vi "Ic_CylindricalLens.vi"(6 "Pixel Pitch 0:20um_or_ 1:12.5um":u8, 7 "Mode Select":enum32{"Row", "Column"}(radio), 8 "error in (no error)":errorcluster, 9 "Wave Length / nm":u32=1064, 10 "Cylindrical Focus / mm":i32=5000, 11 "2D array in (LCOS size buf)":u8[][](array[numeric])) -> (0 "error out":errorcluster, 3 "2D array out":u8[][](array[numeric]))   [LabVIEW 2016]
uses:
  SLM_Control_VI_source/Image_Control.dll
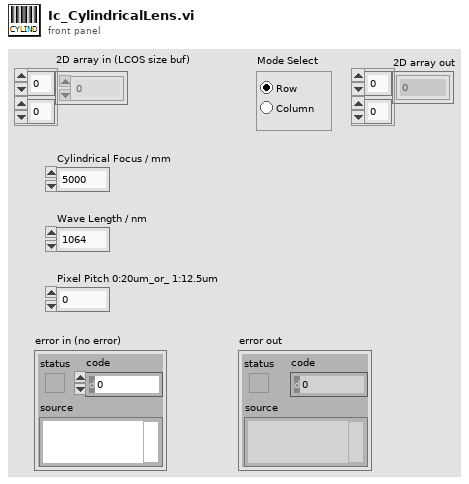
[diagram p1: front panel]
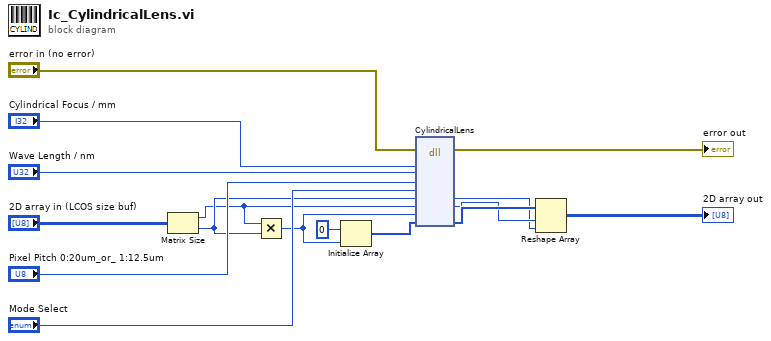
[diagram p0: block diagram]
diagram:
  n1 = Matrix Size(0:"2D array in (LCOS size buf)") -> (1:w9:i32, 2:w10:i32)
  n2 = Multiply(x=w9, y=w10) -> (x*y=w8:i32)
  n3 = Initialize Array(u8 0 ("要素"), w8) -> (w7:u8[])
  n4 = dll-call lib="C:/Users/hs5921/Desktop/SLM_Control_VI_source/Image_Control.dll" fn="CylindricalLens"(error in="error in (no error)", "CylindricalFocusMm"="Cylindrical Focus / mm", "WaveLengthNm"="Wave Length / nm", "PixelPitch0:20um_or_1:1.25um"="Pixel Pitch 0:20um_or_ 1:12.5um", "ModeSelect"="Mode Select", "X_pixel_target"=w10, "Y_pixel_target"=w9, "targetDataSize"=w8, "1DArrayOut"=w7) -> (error out=→"error out":errorcluster, "X_pixel_target"=w4:i32, "Y_pixel_target"=w5:i32, "1DArrayOut"=w6:u8[])  [unwired: 8 in, 1 out]
  n5 = Reshape Array(w6, w5, w4) -> (→"2D array out":u8[][])
